vi "HoppingStep(Nonlinear-XZ-TargetMultilayerImage).vi"() -> ()   [LabVIEW 2014]
uses:
  <vilib>/Platform/TimedLoop/XDataNode/timing_clust.ctl
  <vilib>/Platform/TimedLoop/XDataNode/nitl_modes.ctl
  <vilib>/Platform/TimedLoop/XDataNode/wakeup.ctl
  <vilib>/rvi/Emulation/niFpgaGetClockAttributes.vi
  <vilib>/rvi/Emulation/niFpgaSctlEmulationGetInTimedLoop.vi
  <vilib>/rvi/Emulation/niFpgaEmulationReportErrorSimple.vi
  <vilib>/rvi/eio/common/nirviEmuTemplateMethod_errors.vi
  <vilib>/rvi/Emulation/niFpgaProcessEmulError.vi
  <vilib>/rvi/Emulation/niFpgaCriticalErrorInLSC.vi
  <vilib>/rvi/interface/RandomDataEmulation/niFpgaRandomDataHandleErrors.vi
  <vilib>/eio/EIONode/EIONode.xnode
  <vilib>/Platform/TimedLoop/XDataNode/XDataNode.xnode
  <vilib>/rvi/DataTransferAndStorage/Container/XNode/niFpgaContainer.xnode
  <vilib>/rvi/interface/RandomDataEmulation/nirviRandomDataFpgaReadWriteTemplate.vi
  <vilib>/Platform/TimedLoop/XDataNode/XDNodeRunTimeDep.lvlib
panel:
  in  "ScanLayerNum":u32
  in  "threshold":sgl
  in  "ExtraStepIn":u32
  in  "TimeConstant":u32
  in  "LowPassFilter":i16
  in  "BottomSleep us":i16=80
  in  "UpperSleep us":i16=150
  out "ZRealPos":i16
  in  "RelativeWithdraw":i16
  out "Waveform Chart":i32(graph)
  in  "stop":bool
  out "Z":i32(graph)
  in  "ZOffset":i16
  in  "XOffset":i16
  in  "XNum":i16
  in  "XStepIndex":i16
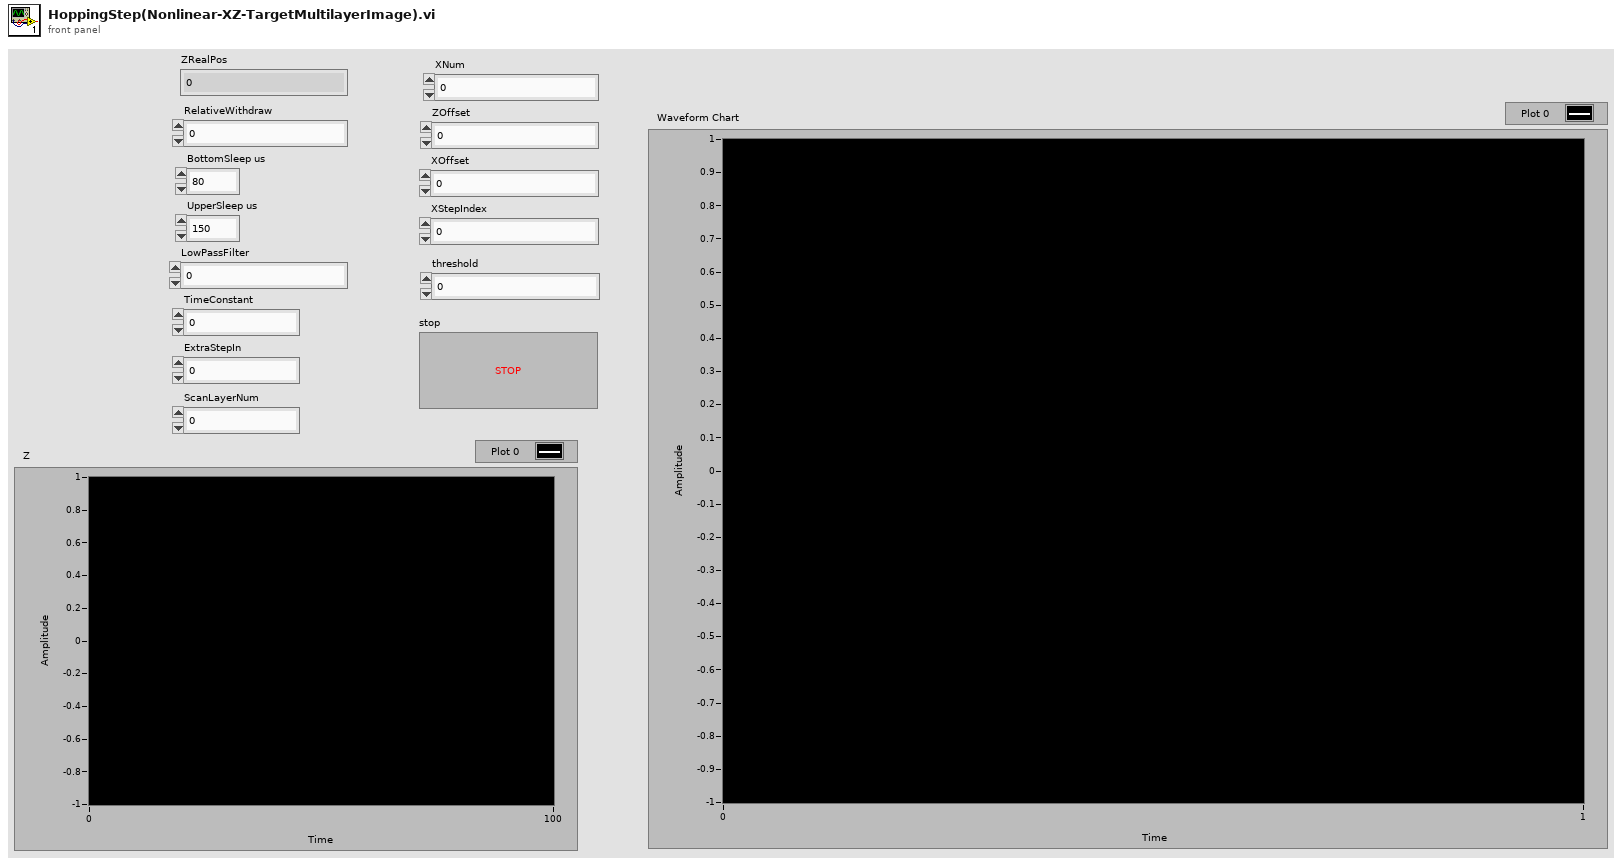
[diagram p1: front panel]
types:
  T1 = typedef "XDNodeRunTimeDep.lvlib/timing_clust.ctl" = cluster{"Expected End [f-1]":u64, "Actual End [f-1]":u64, "Finished Late? [f-1]":bool, "Expected End [i-1]":u64, "Actual End [i-1]":u64, "Finished Late? [i-1]":bool, "Expected Start [i]":u64, "Actual Start [i]":u64, "Expected Start [f]":u64, "Actual Start [f]":u64, "Source Name":string, "Structure Name":string, "Period":i64, "Deadline":i64, "Offset":i64, "Start":i64, "Priority":i32, "Timeout":i32, "Mode":T2, "Wakeup Reason":T3, "Error":errorcluster, "Source Type":string, "Secondary Source Type":string, "Global End Time":u64, "Global Start Time":u64, "Frame Duration":u64, "Iteration Duration":u64, "Assigned CPU":i32, "I/O Scan Engine Mode":u32}
  T2 = typedef "XDNodeRunTimeDep.lvlib/nitl_modes.ctl" = enum32{"No Change", "Process missed periods, maintain original phase", "Discard missed periods, maintain original phase", "Process missed periods, ignore original phase", "Discard missed periods, ignore original phase"}
  T3 = typedef "XDNodeRunTimeDep.lvlib/wakeup.ctl" = enum32{"Normal", "Aborted", "Asynchronous wakeup", "Timing source error", "Timed loop error", "Timeout"}
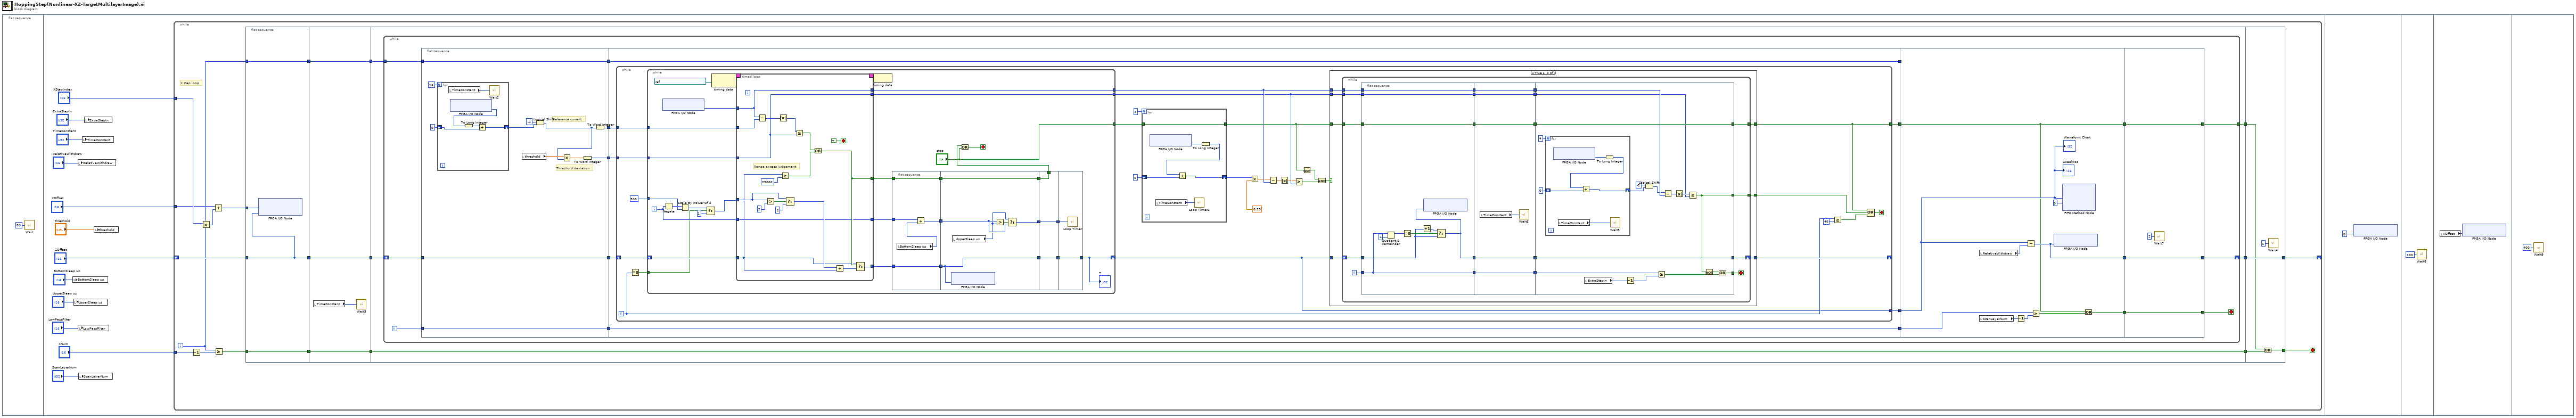
[diagram p0: block diagram]
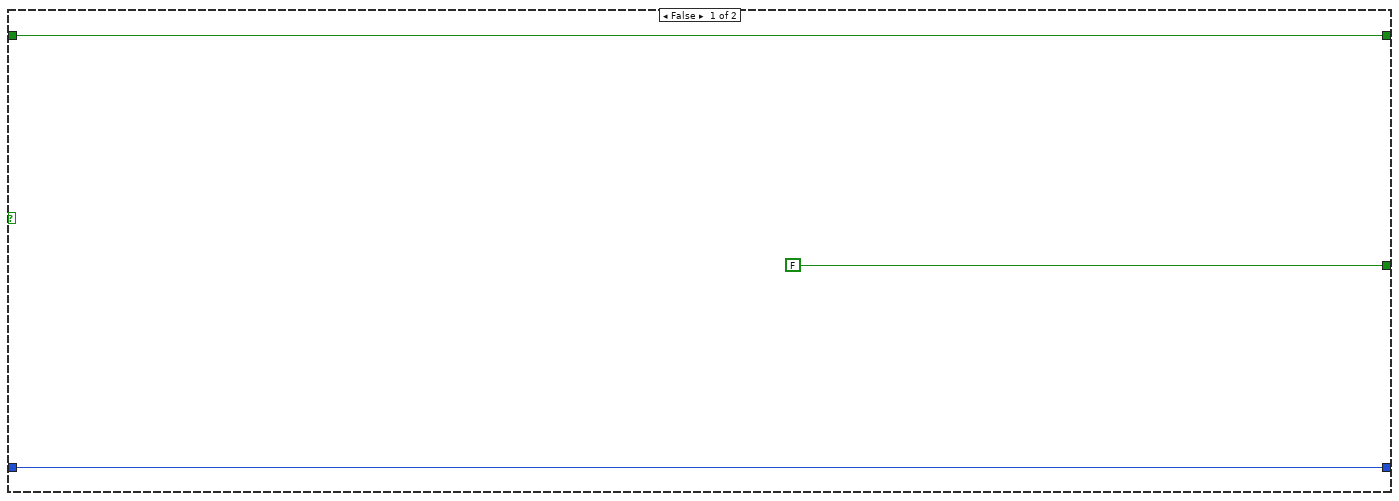
[diagram p2: hidden frame]
diagram:
  n1 = flat-sequence {
    frame #0 {
      n2 = call "Wait"("Count(mSec)"=u32 80 ("Count(uSec)")) -> ()  [unwired: 1 out]
    }
    frame #1 {
      n3 = local write "BottomSleep us"("BottomSleep us") -> ()
      n4 = local write "UpperSleep us"("UpperSleep us") -> ()
      n5 = local write "RelativeWithdraw"("RelativeWithdraw") -> ()
      n6 = local write "LowPassFilter"("LowPassFilter") -> ()
      n7 = local write "ScanLayerNum"("ScanLayerNum") -> ()
      n8 = local write "TimeConstant"("TimeConstant") -> ()
      n9 = local write "ExtraStepIn"("ExtraStepIn") -> ()
      n10 = local write "threshold"("threshold") -> ()
      n11 = while {
        tunnel: "XNum" -> [w27]
        tunnel: "XStepIndex" -> [w28]
        shift-right: [w17] -> _
        shift-left: "ZOffset" -> [w29]
        tunnel: "XOffset" -> [w25]
        i -> [w16]
        stop <- w31 stop-if-true
        # "X step loop"
        n12 = Decrement(x=w27) -> (x-1=w26:i16)
        n13 = Multiply(x=w28, y=w16) -> (x*y=w30:i32)
        n14 = Add(x=w25, y=w30) -> (x+y=w19:i32)
        n15 = Greater Or Equal?(x=w16, y=w26) -> (x >= y?=w23:bool)
        n16 = flat-sequence {
          tunnel: [w37] -> w24
          tunnel: w29 -> [w37]
          tunnel: w23 -> [w36]
          tunnel: [w36] -> w21
          tunnel: w19 -> [w35]
          tunnel: w16 -> [w34]
          tunnel: [w34] -> w14
          tunnel: [w41] -> w33
          tunnel: w24 -> [w41]
          tunnel: [w40] -> w22
          tunnel: w21 -> [w40]
          tunnel: [w38] -> w15
          tunnel: w14 -> [w38]
          tunnel: w33 -> [w46]
          tunnel: [w45] -> w32
          tunnel: w22 -> [w44]
          tunnel: [w44] -> w20
          tunnel: [w43] -> w18
          tunnel: w15 -> [w42]
          tunnel: [w279] -> w17
          tunnel: [w280] -> w31
          tunnel: w18 -> [w279]
          tunnel: w20 -> [w276]
          tunnel: w32 -> [w277]
          frame #0 {
            n17 = xnode "FPGA I/O Node"("Connector0/AO2"=w35, "Connector0/AO0"=w37) -> ()  [unwired: 2 in, 2 out]
          }
          frame #1 {
            n18 = local read "TimeConstant"() -> (w39:u32)
            n19 = call "Wait3"("Count(uSec)"=w39) -> ()  [unwired: 1 out]
          }
          frame #2 {
            n20 = while {
              tunnel: [w60] -> w45
              shift-right: [w57] -> w43
              shift-left: w46 -> [w61]
              tunnel: w42 -> [w52]
              i -> [w56]
              stop <- w53 stop-if-true
              n21 = flat-sequence {
                tunnel: [w72] -> w64
                tunnel: [w73] -> w63
                tunnel: [w76] -> w62
                tunnel: w61 -> [w76]
                tunnel: w56 -> [w69]
                tunnel: [w69] -> w55
                tunnel: w52 -> [w65]
                tunnel: [w65] -> w51
                tunnel: w64 -> [w87]
                tunnel: w63 -> [w86]
                tunnel: w62 -> [w85]
                tunnel: [w88] -> w59
                tunnel: [w84] -> w58
                tunnel: w55 -> [w83]
                tunnel: [w83] -> w54
                tunnel: w51 -> [w82]
                tunnel: [w82] -> w50
                tunnel: w59 -> [w266]
                tunnel: w58 -> [w268]
                tunnel: w54 -> [w262]
                tunnel: w50 -> [_]
                tunnel: [w266] -> w49
                tunnel: [w270] -> w48
                tunnel: [w267] -> w47
                tunnel: [w273] -> w53
                tunnel: [w274] -> w57
                tunnel: [w275] -> w60
                tunnel: w49 -> [w275]
                tunnel: w48 -> [w274]
                tunnel: w47 -> [w273]
                frame #0 {
                  # "Threshold deviation"
                  # "Reference current"
                  n22 = for {
                    N: 16 -> [_]
                    shift-right: [w81] -> w67
                    shift-left: 0 -> [w80]
                    n23 = local read "TimeConstant"() -> (w77:u32)
                    n24 = xnode "FPGA I/O Node"() -> ("Connector0/AI1"=w78:i16)  [unwired: 1 in, 1 out]
                    n25 = To Long Integer(number=w78) -> (32bit integer=w79:i32)
                    n26 = Add(x=w79, y=w80) -> (x+y=w81:i32)
                    n27 = call "Wait2"("Count(uSec)"=w77) -> ()  [unwired: 1 out]
                  }
                  n28 = local read "threshold"() -> (w70:sgl)
                  n29 = Logical Shift(y=i8 -4, x=w67) -> (x << y=w66:i32)
                  n30 = Multiply(x=w70, y=w66) -> (x*y=w74:sgl)
                  n31 = To Word Integer(number=w74) -> (16bit integer=w73:i16)
                  n32 = To Word Integer(number=w66) -> (16bit integer=w72:i16)
                }
                frame #1 {
                  n33 = while {
                    tunnel: [w95] -> w88
                    tunnel: w87 -> [w101]
                    tunnel: w86 -> [w100]
                    shift-right: [w97] -> _
                    shift-left: w85 -> [w98]
                    tunnel: [w89] -> w84
                    i -> [w92]
                    stop <- w96 stop-if-true
                    n34 = Equal To 0?(x=w92) -> (x = 0?=w93:bool)
                    n35 = while {
                      tunnel: w101 -> [w139]
                      tunnel: w100 -> [w141]
                      tunnel: ["stop"] -> w109
                      shift-right: [w122] -> w89
                      shift-left: w98 -> [w136]
                      tunnel: i16 300 -> [w124]
                      tunnel: [w121] -> w113
                      tunnel: [w120] -> w112
                      tunnel: w93 -> [w119]
                      i -> [w123]
                      stop <- w143 stop-if-true
                      n36 = xnode "FPGA I/O Node"() -> ("Connector0/AI1"=w140:i16)  [unwired: 1 in, 1 out]
                      n37 = Negate(x=w123) -> (-x=w125:i32)
                      n38 = Scale By Power Of 2(n=w125, x=w124) -> (x*2^n=w118:i16)
                      n39 = Select(t=w118, s=w119, f=i16 1) -> (s? t:f=w116:i16)
                      n40 = node-c288(refnum<k21> "40 MHz Onboard Clock" ("Source Name")) -> (w146:T1)
                      n41 = timed-loop {
                        timing: w146 -> [_]
                        timing-out: [_] -> w145
                        tunnel: w139 -> [w180]
                        tunnel: w141 -> [w164]
                        tunnel: w140 -> [w163]
                        tunnel: [w176] -> w137
                        tunnel: [w175] -> w135
                        tunnel: w136 -> [w165]
                        tunnel: w116 -> [w168]
                        tunnel: [w170] -> w126
                        tunnel: w123 -> [w170]
                        tunnel: [w164] -> w120
                        tunnel: [w163] -> w121
                        stop <- TRUE stop-if-true
                        # "Range excess judgement"
                        n42 = Subtract(x=w163, y=w180) -> (x-y=w166:i16)
                        n43 = Greater?(x=w168, y=i16 2) -> (0:w167:bool)
                        n44 = Absolute Value(x=w166) -> (abs(x)=w179:i16)
                        n45 = Greater Or Equal?(x=w165, y=i16 29000) -> (x >= y?=w177:bool)
                        n46 = Select(t=w168, s=w167, f=1) -> (s? t:f=w171:i32)
                        n47 = Greater Or Equal?(x=w179, y=w164) -> (x >= y?=w178:bool)
                        n48 = Or(x=w178, y=w177) -> (x .or. y?=w175:bool)
                        n49 = Add(x=w171, y=w165) -> (x+y=w173:i32)
                        n50 = Select(t=w165, s=w175, f=w173) -> (s? t:f=w176:i32)
                      }
                      n51 = node-c288(w145) -> ()
                      n52 = flat-sequence {
                        tunnel: [w151] -> w138
                        tunnel: w137 -> [w151]
                        tunnel: w135 -> [w150]
                        tunnel: [w150] -> w134
                        tunnel: [w148] -> w127
                        tunnel: w126 -> [w149]
                        tunnel: w138 -> [w152]
                        tunnel: [w152] -> w133
                        tunnel: w134 -> [w157]
                        tunnel: [w157] -> w131
                        tunnel: [w155] -> w128
                        tunnel: w127 -> [w154]
                        tunnel: w133 -> [w160]
                        tunnel: [w160] -> w132
                        tunnel: w131 -> [w159]
                        tunnel: [w159] -> w130
                        tunnel: [w158] -> w129
                        tunnel: w128 -> [w158]
                        tunnel: w132 -> [w162]
                        tunnel: [w162] -> w122
                        tunnel: w129 -> [w161]
                        frame #0 {
                          n53 = local read "BottomSleep us"() -> (w147:i16)
                          n54 = Add(x=w149, y=w147) -> (x+y=w148:i32)
                        }
                        frame #1 {
                          n55 = xnode "FPGA I/O Node"("Connector0/AO0"=w152) -> ()  [unwired: 1 in, 1 out]
                          n56 = local read "UpperSleep us"() -> (w153:i16)
                          n57 = Greater?(x=w154, y=w153) -> (0:w156:bool)
                          n58 = Select(t=w153, s=w156, f=w154) -> (s? t:f=w155:i32)
                        }
                        frame #2 {
                        }
                        frame #3 {
                          n59 = call "Loop Timer"("Count(uSec)"=w161) -> ()  [unwired: 1 out]
                        }
                      }
                      n60 = Or(x=w130, y="stop") -> (x .or. y?=w143:bool)
                      "Z" <- w122
                    }
                    n61 = for {
                      N: 4 -> [_]
                      tunnel: w109 -> [w193]
                      tunnel: [w193] -> w114
                      shift-right: [w189] -> w107
                      shift-left: 0 -> [w191]
                      n62 = xnode "FPGA I/O Node"() -> ("Connector0/AI1"=w192:i16)  [unwired: 1 in, 1 out]
                      n63 = local read "TimeConstant"() -> (w188:u32)
                      n64 = call "Loop Timer2"("Count(uSec)"=w188) -> ()  [unwired: 1 out]
                      n65 = To Long Integer(number=w192) -> (32bit integer=w190:i32)
                      n66 = Add(x=w190, y=w191) -> (x+y=w189:i32)
                    }
                    n67 = Multiply(x=w107, y=sgl 0.25) -> (x*y=w106:sgl)
                    n68 = Subtract(x=w106, y=w113) -> (x-y=w105:sgl)
                    n69 = Absolute Value(x=w105) -> (abs(x)=w104:sgl)
                    n70 = Greater Or Equal?(x=w104, y=w112) -> (x >= y?=w103:bool)
                    n71 = Not(x=w114) -> (.not. x?=w102:bool)
                    n72 = And(x=w102, y=w103) -> (x .and. y?=w115:bool)
                    n73 = case shown="True" w115 {
                      tunnel: w114 -> [w196 w203]
                      tunnel: [w196 w202] -> w95
                      tunnel: w113 -> [_ w201]
                      tunnel: w112 -> [_ w200]
                      tunnel: w89 -> [w195 w199]
                      tunnel: [w195 w198] -> w97
                      tunnel: [FALSE w197] -> w94
                      frame False {
                      }
                      frame True {
                        n74 = while {
                          tunnel: w201 -> [w212]
                          tunnel: w200 -> [w211]
                          tunnel: [w208] -> w197
                          shift-right: [w209] -> w198
                          shift-left: w199 -> [w210]
                          tunnel: w203 -> [w214]
                          tunnel: [w213] -> w202
                          i -> [w206]
                          stop <- w204 stop-if-true
                          n75 = flat-sequence {
                            tunnel: w211 -> [w230]
                            tunnel: w212 -> [w231]
                            tunnel: w214 -> [w232]
                            tunnel: [w232] -> w222
                            tunnel: [w231] -> w221
                            tunnel: [w230] -> w220
                            tunnel: w210 -> [w224]
                            tunnel: [w223] -> w219
                            tunnel: [w229] -> w207
                            tunnel: w206 -> [w229]
                            tunnel: [w238] -> w218
                            tunnel: [w237] -> w217
                            tunnel: [w236] -> w216
                            tunnel: w222 -> [w238]
                            tunnel: w221 -> [w237]
                            tunnel: w220 -> [w236]
                            tunnel: [w235] -> w215
                            tunnel: w219 -> [w235]
                            tunnel: w207 -> [w233]
                            tunnel: [w233] -> w205
                            tunnel: w218 -> [w256]
                            tunnel: [w256] -> w213
                            tunnel: w217 -> [w251]
                            tunnel: w216 -> [w250]
                            tunnel: w215 -> [w249]
                            tunnel: [w249] -> w209
                            tunnel: [w243] -> w208
                            tunnel: w205 -> [w248]
                            tunnel: [w244] -> w204
                            frame #0 {
                              n76 = Quotient & Remainder(x=w229, y=4) -> (x-y*floor(x/y)=w227:i32)  [unwired: 1 out]
                              n77 = Equal To 0?(x=w227) -> (x = 0?=w226:bool)
                              n78 = Increment(x=w224) -> (x+1=w225:i32)
                              n79 = Select(t=w225, s=w226, f=w224) -> (s? t:f=w223:i32)
                              n80 = xnode "FPGA I/O Node"("Connector0/AO0"=w223) -> ()  [unwired: 1 in, 1 out]
                            }
                            frame #1 {
                              n81 = local read "TimeConstant"() -> (w234:u32)
                              n82 = call "Wait6"("Count(uSec)"=w234) -> ()  [unwired: 1 out]
                            }
                            frame #2 {
                              n83 = for {
                                N: 4 -> [_]
                                shift-right: [w258] -> w240
                                shift-left: 0 -> [w260]
                                n84 = xnode "FPGA I/O Node"() -> ("Connector0/AI1"=w261:i16)  [unwired: 1 in, 1 out]
                                n85 = local read "TimeConstant"() -> (w257:u32)
                                n86 = To Long Integer(number=w261) -> (32bit integer=w259:i32)
                                n87 = Add(x=w259, y=w260) -> (x+y=w258:i32)
                                n88 = call "Wait5"("Count(uSec)"=w257) -> ()  [unwired: 1 out]
                              }
                              n89 = local read "ExtraStepIn"() -> (w247:u32)
                              n90 = Decrement(x=w247) -> (x-1=w246:u32)
                              n91 = Logical Shift(y=i8 -2, x=w240) -> (x << y=w239:i32)
                              n92 = Greater Or Equal?(x=w248, y=w246) -> (x >= y?=w245:bool)
                              n93 = Subtract(x=w239, y=w251) -> (x-y=w253:i32)
                              n94 = Absolute Value(x=w253) -> (abs(x)=w252:i32)
                              n95 = Greater Or Equal?(x=w252, y=w250) -> (x >= y?=w243:bool)
                              n96 = Not(x=w243) -> (.not. x?=w242:bool)
                              n97 = Or(x=w242, y=w245) -> (x .or. y?=w244:bool)
                            }
                          }
                        }
                      }
                    }
                    n98 = Greater Or Equal?(x=w92, y=40) -> (x >= y?=w90:bool)
                    n99 = Compound Arithmetic op=OR(w95, w94, w90) -> (w96:bool)
                  }
                }
                frame #2 {
                  n100 = local read "RelativeWithdraw"() -> (w271:i16)
                  n101 = local read "ScanLayerNum"() -> (w264:u32)
                  n102 = Decrement(x=w264) -> (x-1=w263:u32)
                  n103 = Subtract(x=w268, y=w271) -> (x-y=w270:i32)
                  n104 = Greater Or Equal?(x=w262, y=w263) -> (x >= y?=w265:bool)
                  n105 = xnode "FPGA I/O Node"("Connector0/AO0"=w270) -> ()  [unwired: 1 in, 1 out]
                  n106 = xnode ("FIFO Method Node")("Element"=w268, "Timeout"=0) -> ()  [unwired: 1 in, 2 out]
                  n107 = Or(x=w266, y=w265) -> (x .or. y?=w267:bool)
                  "Waveform Chart" <- w268
                  "ZRealPos" <- w268
                }
                frame #3 {
                  n108 = call "Wait7"("Count(mSec)"=u32 2) -> ()  [unwired: 1 out]
                }
              }
            }
          }
          frame #3 {
            n109 = Or(x=w277, y=w276) -> (x .or. y?=w280:bool)
            n110 = call "Wait4"("Count(mSec)"=u32 1) -> ()  [unwired: 1 out]
          }
        }
      }
    }
    frame #2 {
      n111 = xnode "FPGA I/O Node"("Connector0/AO0"=i16 0) -> ()  [unwired: 1 in, 1 out]
    }
    frame #3 {
      n112 = call "Wait8"("Count(uSec)"=u32 200) -> ()  [unwired: 1 out]
    }
    frame #4 {
      n113 = local read "XOffset"() -> (w283:i16)
      n114 = xnode "FPGA I/O Node"("Connector0/AO2"=w283) -> ()  [unwired: 1 in, 1 out]
    }
    frame #5 {
      n115 = call "Wait9"("Count(uSec)"=u32 400) -> ()  [unwired: 1 out]
    }
  }
